vi "PI-Move PIFOC.vi"(8 "error in (no error)":errorcluster, 11 "params":variant) -> (0 "error out":errorcluster, 3 "PIFOC out":T1={"PIFOC Position (mm) [SET]"=0.0, "PIFOC Position\n(um) [ACT]"=0.0087, "last command"=""} {"PIFOC Position\n(um) [ACT]" format="%.2f"; "PIFOC Position (mm) [SET]" min=0.0 max=100.0 step=0.1 scale=0.0..100.0})   [LabVIEW 2020]
uses:
  _Controls/PIFOC Position.ctl
  SDK/GCS_LabVIEW_digital/Low Level/Communication.llb/Global1.vi
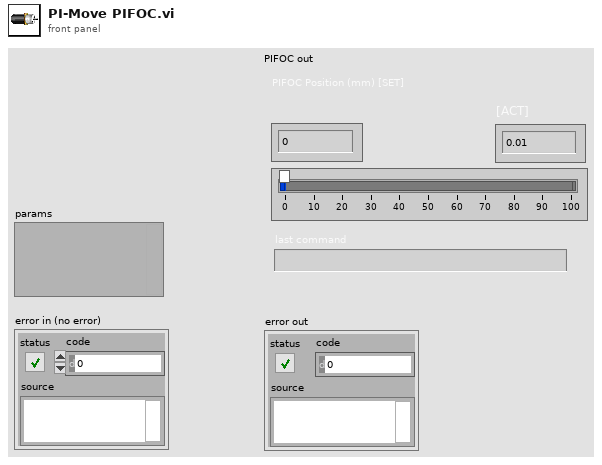
[diagram p1: front panel]
types:
  T1 = typedef "PIFOC Position.ctl" = cluster{"PIFOC Position (mm) [SET]":dbl, "PIFOC Position\n(um) [ACT]":dbl, "last command":string}
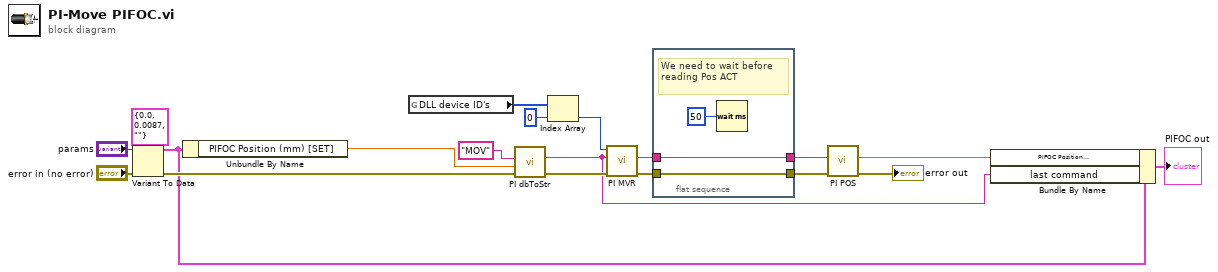
[diagram p0: block diagram]
diagram:
  n1 = Variant To Data(error in="error in (no error)", type=T1 {"PIFOC Position (mm) [SET]"=0.0, "PIFOC Position\n(um) [ACT]"=0.0087, "last command"=""} ("NewVal"), Variant="params") -> (data=w4:T1, error out=w18:errorcluster)
  n2 = Unbundle By Name(w4) -> ("PIFOC Position (mm) [SET]"=w5:dbl)
  n3 = global read "Global1.vi" "DLL device ID's"() -> (w14:i32[])
  n4 = call "PI dbToStr.vi"("Start"=w5, "String in"="MOV") -> ("String out"=w2:string)  [unwired: 9 in]
  n5 = Index Array(array=w14, index=0) -> (element=w7:i32)
  n6 = call "PI MVR.vi"("error in (no error)"=w18, "String"=w2, "PI ID in"=w7) -> ("error out"=w12:errorcluster, "szCommand"=w10:string)  [unwired: 6 in, 1 out]
  n7 = flat-sequence {
    tunnel: w12 -> [w21]
    tunnel: [w21] -> w13
    tunnel: w10 -> [w19]
    tunnel: [w19] -> w9
    frame #0 {
      # "We need to wait before reading Pos ACT"
      n8 = Wait (ms)(milliseconds to wait=u32 50 ("Post Wait")) -> ()  [unwired: 1 out]
    }
  }
  n9 = call "PI POS.vi"("error in (no error)"=w13, "query"=w9) -> ("error out"=→"error out":errorcluster, "Position"=w3:dbl)  [unwired: 7 in, 1 out]
  n10 = Bundle By Name(cluster=w4, "PIFOC Position\n(um) [ACT]"=w3, "last command"=w2) -> (→"PIFOC out":T1)
